vi "psychophysics.vi"() -> ()   [LabVIEW 2017]
panel:
  out "XY Graph":cluster{dbl[], dbl[]}[](graph)
  in  "N":u32(knob) scale=0.0..100.0
  in  "?":bool
  in  "outer":dbl=6.0 format="%#_13g"
  in  "inner":dbl=2.0 format="%#_13g"
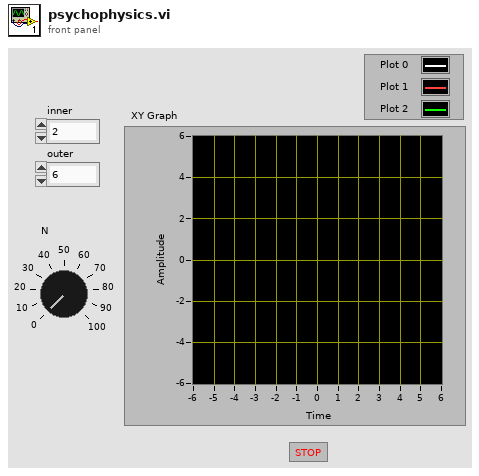
[diagram p1: front panel]
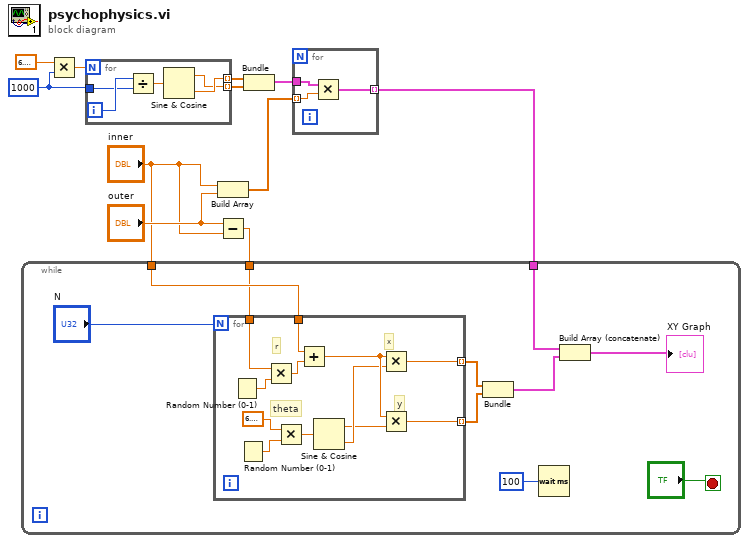
[diagram p0: block diagram]
diagram:
  w5 = 1000
  n1 = Multiply(x=6.283185307179586, y=w5) -> (x*y=w6:dbl)
  n2 = for {
    N: w6 -> [_]
    tunnel: [w16] -> w9 mode=indexing
    tunnel: [w15] -> w8 mode=indexing
    tunnel: w5 -> [w13]
    i -> [w14]
    n3 = Divide(x=w14, y=w13) -> (x/y=w12:dbl)
    n4 = Sine & Cosine(0:w12) -> (1:w15:dbl, 2:w16:dbl)
  }
  n5 = Build Array("inner", "outer") -> (w10:dbl[])
  n6 = Subtract(x="outer", y="inner") -> (x-y=w1:dbl)
  n7 = Bundle(w9, w8) -> (w7:cluster{dbl[], dbl[]})  [unwired: 1 in]
  n8 = for {
    tunnel: w10 -> [w19] mode=indexing
    tunnel: [w18] -> w3 mode=indexing
    tunnel: w7 -> [w17]
    n9 = Multiply(x=w17, y=w19) -> (x*y=w18:cluster{dbl[], dbl[]})
  }
  n10 = while {
    tunnel: w3 -> [w27]
    tunnel: "inner" -> [w25]
    tunnel: w1 -> [w24]
    stop <- "?" stop-if-true
    n11 = for {
      N: "N" -> [_]
      tunnel: w25 -> [w33]
      tunnel: w24 -> [w32]
      tunnel: [w31] -> w23 mode=indexing
      tunnel: [w30] -> w22 mode=indexing
      # "r"
      # "theta"
      # "x"
      # "y"
      n12 = Random Number (0-1)() -> (number: 0 to 1=w35:dbl)
      n13 = Random Number (0-1)() -> (number: 0 to 1=w37:dbl)
      n14 = Multiply(x=w32, y=w35) -> (x*y=w36:dbl)
      n15 = Multiply(x=6.283185307179586, y=w37) -> (x*y=w38:dbl)
      n16 = Add(x=w33, y=w36) -> (x+y=w41:dbl)
      n17 = Sine & Cosine(0:w38) -> (1:w39:dbl, 2:w40:dbl)
      n18 = Multiply(x=w41, y=w40) -> (x*y=w31:dbl)
      n19 = Multiply(x=w41, y=w39) -> (x*y=w30:dbl)
    }
    n20 = Bundle(w23, w22) -> (w21:cluster{dbl[], dbl[]})  [unwired: 1 in]
    n21 = Wait (ms)(milliseconds to wait=u32 100 ("millisecond timer value")) -> ()  [unwired: 1 out]
    n22 = Build Array (concatenate)(w27, w21) -> (→"XY Graph":cluster{dbl[], dbl[]}[])
  }
